vi "REPLACE.vi"(11 "Dev Actor in":refnum<class "Dev Actor.lvclass">) -> (2 "Destroy?":bool, 3 "Dev Actor out":refnum<class "Dev Actor.lvclass">)   [LabVIEW 2021, in "Dev Actor.lvlib" / "Dev Actor.lvclass"]
uses:
  Dev Actor.lvclass
  Dev Actor.lvclass/Dev Actor.ctl
  <vilib>/jettl/jettl/Actor/Actor/Actor.lvclass
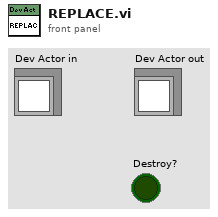
[diagram p1: front panel]
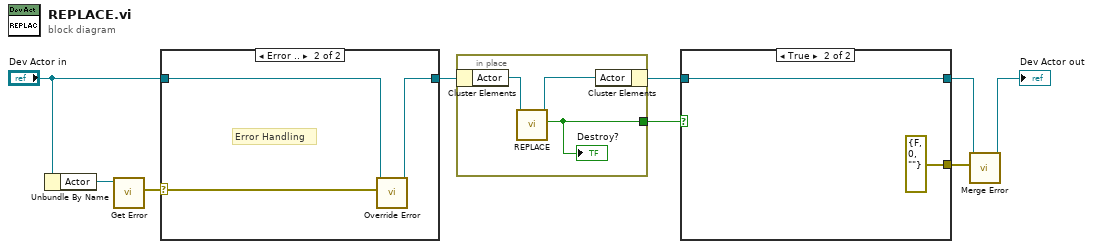
[diagram p0: block diagram]
diagram:
  n1 = Unbundle By Name("Dev Actor in") -> ("Actor"=w5:refnum<class "Actor.lvclass">)
  n2 = call-dynamic "Get Error.vi"("Actor in"=w5) -> ("Error"=w6:errorcluster)  [unwired: 10 in]
  n3 = case shown="Error .." w6 {
    selector: w6 -> [_ w11]
    tunnel: "Dev Actor in" -> [w10 w13]
    tunnel: [w10 w12] -> w1
    frame No Error {
    }
    frame Error {
      # "Error Handling"
      n4 = call-dynamic "Override Error.vi"("Error"=w11, "Dev Actor in"=w13) -> ("Dev Actor out"=w12:refnum<class "Dev Actor.lvclass">)  [unwired: 9 in]
    }
  }
  n5 = in-place {
    in-place-border: [w14] -> w9
    n6 = in-place-cluster #1(w1) -> ("Actor"=w16:refnum<class "Actor.lvclass">)
    n7 = call-dynamic "REPLACE.vi"("Actor in"=w16) -> ("Destroy?"=w14:bool, "Actor out"=w15:refnum<class "Actor.lvclass">)  [unwired: 9 in]
    "Destroy?" <- w14
    n8 = in-place-cluster #1("Actor"=w15) -> (w3:refnum<class "Dev Actor.lvclass">)
  }
  n9 = case shown="True" w9 {
    tunnel: [_ errorcluster {"status"=FALSE, "code"=0, "source"=""} ("error out")] -> w7
    tunnel: [w17 w19] -> w4
    tunnel: w3 -> [w17 w19]
    frame False {
    }
    frame True {
    }
  }
  n10 = call-dynamic "Merge Error.vi"("Error"=w7, "Dev Actor in"=w4) -> ("Dev Actor out"=→"Dev Actor out":refnum<class "Dev Actor.lvclass">)  [unwired: 9 in]
